vi "Alicat Dynamic Data Example.vi"() -> ()   [LabVIEW 2016]
panel:
  in  "End Program":bool
  out "Dynamic Data":T1
  in  "Minimum time \nbetween readings [ms]":u32
  out "Measurements\nper second":dbl
  in  "COM Port Settings":T2={"Unit ID"="A", "Baud Rate"=enum."19200", "VISA Sesssion In"="COM1"}
  # "This example VI only works with software version 6v0 and above. If using an Alicat with older software, please use the non-dynamic versions of the data collection VI's"
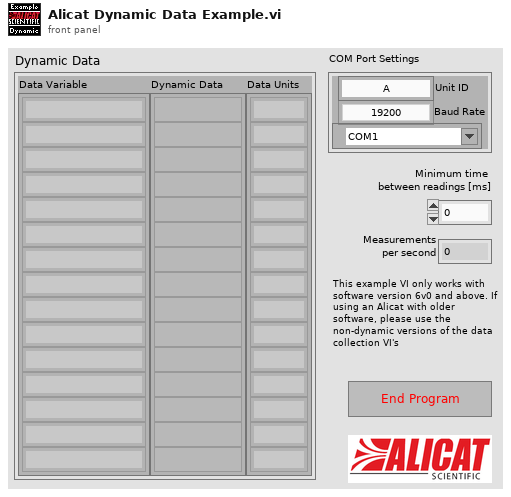
[diagram p1: front panel]
types:
  T1 = cluster{"Data Variable":string[], "Dynamic Data":variant[], "Data Units":string[]}
  T2 = cluster{"Unit ID":string, "Baud Rate":enum8{"2400", "9600", "19200", "38400", "57600", "115200", "Unknown"}, "VISA Sesssion In":refnum<visa-resource-name>}
  T3 = cluster{"Data Variable":string[], "Data Units":string[], "Data is String":bool[]}
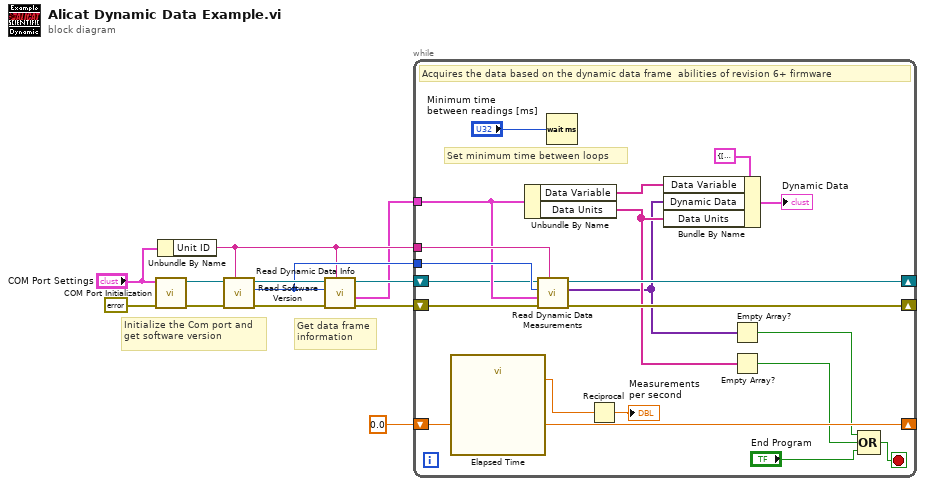
[diagram p0: block diagram]
diagram:
  # "Get data frame\ninformation"
  # "Initialize the Com port and get software version"
  n1 = call "COM Port Initialization.vi"("error in (no error)"=errorcluster {"status"=FALSE, "code"=0, "source"=""}, "Communication Settings"="COM Port Settings") -> ("error out"=w8:errorcluster, "VISA Session Out"=w9:refnum<visa-resource-name>)  [unwired: 8 in]
  n2 = Unbundle By Name("COM Port Settings") -> ("Unit ID"=w2:string)
  n3 = call "Read Software Version.vi"("Unit ID (A)"=w2, "error in"=w8, "VISA Session In"=w9) -> ("error out"=w4:errorcluster, "Software Version"=w3:u8, "VISA Session Out"=w5:refnum<visa-resource-name>)  [unwired: 6 in]
  n4 = call "Read Dynamic Data Info.vi"("Unit ID (A)"=w2, "error in"=w4, "Software Rev"=w3, "VISA Session In"=w5) -> ("error out"=w7:errorcluster, "Dynamic Data Info"=w1:T3, "VISA Session Out"=w6:refnum<visa-resource-name>)  [unwired: 5 in]
  n5 = while {
    shift-right: [w30] -> _
    shift-left: 0.0 ("Set Start Time (s)") -> [w31]
    tunnel: w3 -> [w28]
    tunnel: w2 -> [w29]
    shift-right: [w27] -> _
    shift-left: w6 -> [w20]
    shift-right: [w26] -> _
    shift-left: w7 -> [w19]
    tunnel: w1 -> [w21]
    stop <- w15 stop-if-true
    # "Set minimum time between loops"
    # "Acquires the data based on the dynamic data frame  abilities of revision 6+ firmware"
    n6 = call "Elapsed Time"("Set Start Time (s)"=w31) -> ("Get Start Time (s)"=w30:dbl, "Elapsed Time (s)"=w32:dbl)  [unwired: 11 in, 6 out]
    n7 = Unbundle By Name(w21) -> ("Data Variable"=w22:string[], "Data Units"=w18:string[])
    n8 = call "Read Dynamic Data Measurements.vi"("Unit ID (A)"=w29, "error in"=w19, "Dynamic Data Info"=w21, "Software Rev"=w28, "VISA Session In"=w20) -> ("error out"=w26:errorcluster, "Dynamic Data"=w14:variant[], "VISA Session Out"=w27:refnum<visa-resource-name>)  [unwired: 4 in]
    n9 = Wait (ms)(milliseconds to wait="Minimum time \nbetween readings [ms]") -> ()  [unwired: 1 out]
    n10 = Reciprocal(x=w32) -> (1/x=→"Measurements\nper second":dbl)
    n11 = Bundle By Name(cluster=T1 {"Data Variable"=[], "Dynamic Data"=[], "Data Units"=[]} ("Dynamic Data"), "Data Variable"=w22, "Dynamic Data"=w14, "Data Units"=w18) -> (→"Dynamic Data":T1)
    n12 = Empty Array?(array=w14) -> (empty?=w13:bool)
    n13 = Empty Array?(array=w18) -> (empty?=w16:bool)
    n14 = Compound Arithmetic op=OR(w13, w16, "End Program") -> (w15:bool)
  }
